vi "Set Gate Delay.vi"(8 "error in (no error)":errorcluster, 9 "Delay (Def: 0 s)":dbl, 10 "Gate (Def: A)":T1, 11 "VISA resource name":refnum<visa-resource-name>) -> (0 "error out":errorcluster, 3 "VISA resource name out":refnum<visa-resource-name>)   [LabVIEW 2015, in "SR400.lvlib"]
doc: "GD i { ,t }\nThe GD command sets and reads the gate delays.\ni=0 or 1 designates A gate or B gate and is\nrequired. If t is included, the selected gate delay is\nset to t seconds where 0 <= t <= 999.2E-3. The\nresolution is variable depending upon the 4 most\nsignificant digits of t.\n4 most significant digits resolution in 4th digit\n1000 to 2048 1 (1001,1002,1003,...)\n2048 to 4096 2\n4096 to 8192 4\n8192 to 9992 8 (8192,8200,8208,...)\nFor example, near 10.00 ìs, the allowed values of\nt are 9.984 ìs, 9.992 ìs, 10.00 ìs, 10.01 ìs, etc.\nBelow 1.000 ìs, the resolution is 1 ns. Almost any\nvalue of t may be sent and the SR400 will round to\nthe nearest allowed value. If t is absent, the\nselected gate delay is returned. The gate delay may\nbe set and read regardless of the gate mode. If the\nmode is CW, the gate remains continuous. If the\nmode is SCAN, the GD command sets and reads\nthe starting position of the gate delay. Changing\nthe delay during a scan will cause the delay to be\nset to the new value on the next count period. Note\nthat the scan is not reset. Reading the delay during\na scan always returns the starting delay, not the\ncurrent delay."
uses:
  SR400.lvlib
  Typedefs/Gate.ctl
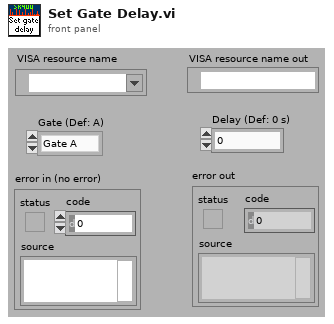
[diagram p1: front panel]
types:
  T1 = typedef "SR400.lvlib/Gate.ctl" = enum16{"Gate A", "Gate B"}
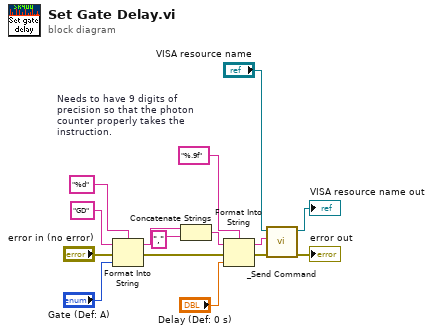
[diagram p0: block diagram]
diagram:
  w8 = "%.9f"  # Needs to have 9 digits of precision so that the photon counter properly takes the instruction.
  n1 = Format Into String(format string="%d", initial string="GD" ("command"), error in="error in (no error)", "Gate (Def: A)") -> (resulting string=w6:string, error out=w7:errorcluster)
  n2 = Concatenate Strings(w6, "," ("command")) -> (w10:string)
  n3 = Format Into String(format string=w8, initial string=w10, error in=w7, "Delay (Def: 0 s)") -> (resulting string=w4:string, error out=w3:errorcluster)
  n4 = call "_Send Command.vi"("error in (no error)"=w3, "Command"=w4, "VISA resource name"="VISA resource name") -> ("error out"=→"error out":errorcluster, "VISA resource name out"=→"VISA resource name out":refnum<visa-resource-name>)  [unwired: 1 in, 6 out]
